vi "Insert Key Value Pair (Single).vi"(8 "error in (no error)":errorcluster, 9 "value":refnum<class "JSON Datatype.lvclass">, 10 "key":string, 11 "JSON Object in":refnum<class "JSON Object.lvclass">) -> (0 "error out":errorcluster, 3 "JSON Object out":refnum<class "JSON Object.lvclass">)   [LabVIEW 2017, in "LVJSON.lvlib" / "JSON Object.lvclass"]
uses:
  JSON Object.lvclass
  JSON Datatype/JSON Datatype.lvclass
  JSON Object.lvclass/JSON Object.ctl
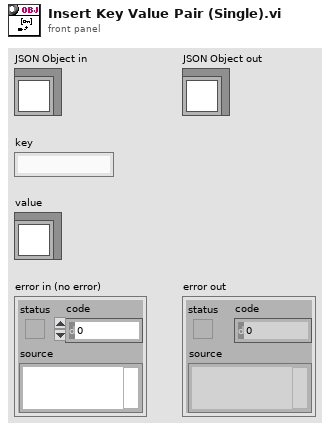
[diagram p1: front panel]
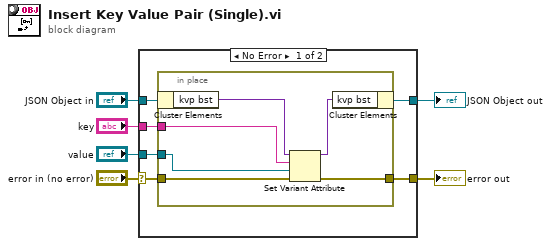
[diagram p0: block diagram]
diagram:
  n1 = case shown="No Error" "error in (no error)" {
    selector: "error in (no error)" -> [w8 w20]
    tunnel: [w7 w20] -> w5
    tunnel: [w11 w19] -> w3
    tunnel: "JSON Object in" -> [w12 w19]
    tunnel: "key" -> [w10 _]
    tunnel: "value" -> [w9 _]
    frame No Error {
      n2 = in-place {
        in-place-border: w10 -> [w17]
        in-place-border: w9 -> [w13]
        in-place-border: w8 -> [w15]
        in-place-border: [w14] -> w7
        n3 = in-place-cluster #1(w12) -> ("kvp bst"=w18:variant)
        n4 = Set Variant Attribute(Variant=w18, name=w17, value=w13, error in=w15) -> (Variant out=w16:variant, error out=w14:errorcluster)  [unwired: 1 out]
        n5 = in-place-cluster #1("kvp bst"=w16) -> (w11:refnum<class "JSON Object.lvclass">)
      }
    }
    frame Error {
    }
  }
  "error out" <- w5
  "JSON Object out" <- w3
